vi "Agilent PWM Configure Serial Port.vi"(8 "error in (no error)":errorcluster, 11 "VISA Resource Name":refnum<visa-resource-name>) -> (0 "error out":errorcluster, 3 "dup VISA Resource Name":refnum<visa-resource-name>)   [LabVIEW 2011]
panel:
  in  "Baud Rate":T1(ring)
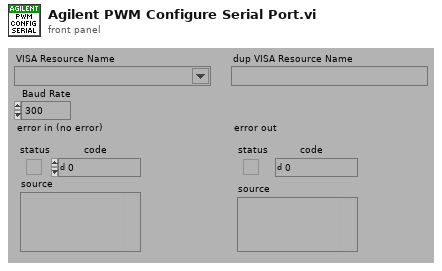
[diagram p1: front panel]
types:
  T1 = enum32{"300", "600", "1200", "2400", "4800", "9600"}
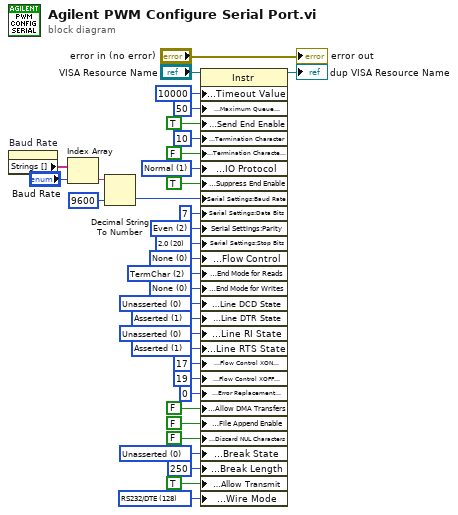
[diagram p0: block diagram]
diagram:
  w33 = i16 128 items=["Unknown"=-1, "RS485/Wire4"=0, "RS485/Wire2-EchoDTR"=1, "RS485/Wire2-CtrlDTR"=2, "RS485/Wire2-Auto"=3, "RS232/DTE"=128, "RS232/DCE"=129, "RS232/AUTO"=130] ("Serial Settings:Wire Mode")
  w30 = i16 0 items=["Unknown"=-1, "Unasserted"=0, "Asserted"=1] ("Modem Line Settings:Break State")
  w23 = i16 1 items=["Unknown"=-1, "Unasserted"=0, "Asserted"=1] ("Modem Line Settings:Line RTS State")
  w22 = i16 0 items=["Unknown"=-1, "Unasserted"=0, "Asserted"=1] ("Modem Line Settings:Line RI State")
  w21 = i16 1 items=["Unknown"=-1, "Unasserted"=0, "Asserted"=1] ("Modem Line Settings:Line DTR State")
  w20 = i16 0 items=["Unknown"=-1, "Unasserted"=0, "Asserted"=1] ("Modem Line Settings:Line DCD State")
  w19 = u16 0 items=["None", "LastBit", "TermChar", "Break"] ("Serial Settings:Serial End Mode for Writes")
  w18 = u16 2 items=["None", "LastBit", "TermChar"] ("Serial Settings:Serial End Mode for Reads")
  w17 = u16 0 items=["None", "XON/XOFF", "RTS/CTS", "XON/XOFF & RTS/CTS", "DTR/DSR", "XON/XOFF & DTR/DSR"] ("Serial Settings:Serial Flow Control")
  w16 = u16 20 items=["1.0"=10, "1.5"=15, "2.0"=20] ("Serial Settings:Serial Stop Bits")
  w15 = u16 2 items=["None", "Odd", "Even", "Mark", "Space"] ("Serial Settings:Serial Parity")
  w13 = u16 1 items=["Normal"=1, "VXI/FDC"=2, "GPIB/HS488"=3, "Serial-TCPIP-USB/488-Strings"=4, "USBTMC/Vendor-Specific"=5] ("Message Based Settings:IO Protocol")
  n1 = property on="Baud Rate" class="Enum (strict)"() -> ("Strings []"=w5:string[])  [unwired: 2 in, 2 out]
  n2 = Index Array(array=w5, index="Baud Rate") -> (element=w2:string)
  n3 = Decimal String To Number(string=w2, default (0L)=u32 9600 ("Serial Settings:Serial Data Bits")) -> (number=w1:u32)  [unwired: 1 in, 1 out]
  n4 = property class="Instr"(reference="VISA Resource Name", "General Settings:Timeout Value"=u32 10000, "General Settings:Maximum Queue Length"=u32 50, "Message Based Settings:Send End Enable"=TRUE, "Message Based Settings:Termination Character"=u8 10, "Message Based Settings:Termination Character Enable"=FALSE, "Message Based Settings:IO Protocol"=w13, "Message Based Settings:Suppress End Enable"=TRUE, "Serial Settings:Baud Rate"=w1, "Serial Settings:Data Bits"=u16 7 ("Serial Settings:Serial Data Bits"), "Serial Settings:Parity"=w15, "Serial Settings:Stop Bits"=w16, "Serial Settings:Flow Control"=w17, "Serial Settings:End Mode for Reads"=w18, "Serial Settings:End Mode for Writes"=w19, "Serial Settings:Modem Line Settings:Line DCD State"=w20, "Serial Settings:Modem Line Settings:Line DTR State"=w21, "Serial Settings:Modem Line Settings:Line RI State"=w22, "Serial Settings:Modem Line Settings:Line RTS State"=w23, "Serial Settings:Flow Control XON Character"=u8 17, "Serial Settings:Flow Control XOFF Character"=u8 19, "Serial Settings:Error Replacement Character"=u8 0, "General Settings:Allow DMA Transfers"=FALSE, "Message Based Settings:File Append Enable"=FALSE, "Serial Settings:Discard NUL Characters"=FALSE, "Serial Settings:Modem Line Settings:Break State"=w30, "Serial Settings:Break Length"=i16 250, "Serial Settings:Allow Transmit"=TRUE, "Serial Settings:Wire Mode"=w33) -> (reference out=→"dup VISA Resource Name":refnum<visa-resource-name>)  [unwired: 1 in, 1 out]
  "error out" <- "error in (no error)"
